vi "ConvertDtoY.vi"(8 "error in":errorcluster, 10 "Wiring Configuration":string, 11 "voltage waveform":waveform(dbl)[](array[waveform])) -> (0 "error out":errorcluster, 3 "phase voltage waveform":waveform(dbl)[](array[waveform]))   [LabVIEW 2017, in "McsaAnalysisFunctions.lvlib"]
uses:
  <vilib>/addons/InsightCM/Utilities/Analysis/MCSA/McsaAnalysisFunctions.lvlib
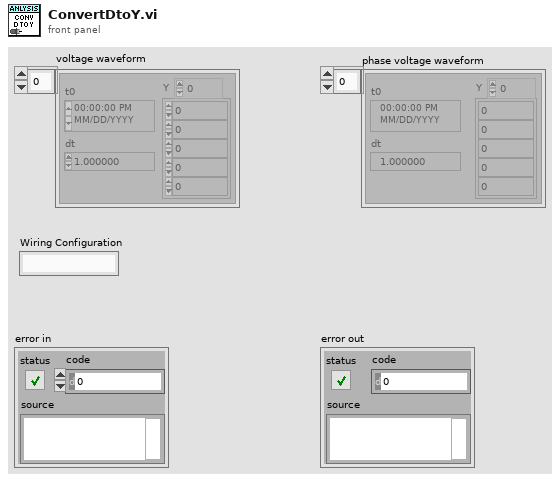
[diagram p1: front panel]
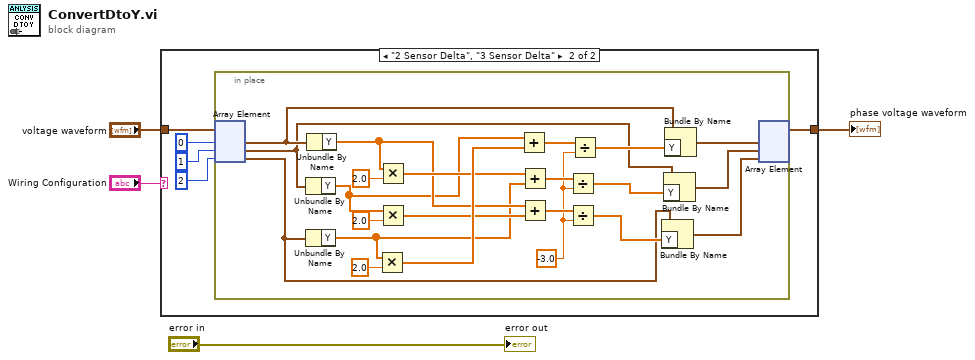
[diagram p0: block diagram]
diagram:
  n1 = case shown="\"2 Sensor Delta\", \"3 Sensor Delta\"" "Wiring Configuration" {
    tunnel: "voltage waveform" -> [w5 w10]
    tunnel: [w5 w9] -> w4
    frame "2 Sensor Wye", "3 Sensor Wye", Default {
    }
    frame "2 Sensor Delta", "3 Sensor Delta" {
      n2 = in-place {
        w17 = -3.0 ("y")
        n3 = in-place-array #1(w10, 0, 1, 2) -> (w16:waveform(dbl), w15:waveform(dbl), w14:waveform(dbl))
        n4 = Unbundle By Name(w15) -> ("Y"=w25:dbl[])
        n5 = Unbundle By Name(w14) -> ("Y"=w24:dbl[])
        n6 = Unbundle By Name(w16) -> ("Y"=w26:dbl[])
        n7 = Multiply(x=w24, y=2.0) -> (x*y=w29:dbl[])
        n8 = Multiply(x=w26, y=2.0) -> (x*y=w28:dbl[])
        n9 = Multiply(x=w25, y=2.0) -> (x*y=w27:dbl[])
        n10 = Add(x=w25, y=w29) -> (x+y=w23:dbl[])
        n11 = Add(x=w28, y=w24) -> (x+y=w22:dbl[])
        n12 = Add(x=w26, y=w27) -> (x+y=w21:dbl[])
        n13 = Divide(x=w22, y=w17) -> (x/y=w19:dbl[])
        n14 = Divide(x=w21, y=w17) -> (x/y=w18:dbl[])
        n15 = Divide(x=w23, y=w17) -> (x/y=w20:dbl[])
        n16 = Bundle By Name(cluster=w14, "Y"=w18) -> (w11:waveform(dbl))
        n17 = Bundle By Name(cluster=w15, "Y"=w19) -> (w12:waveform(dbl))
        n18 = Bundle By Name(cluster=w16, "Y"=w20) -> (w13:waveform(dbl))
        n19 = in-place-array #1(w13, w12, w11) -> (w9:waveform(dbl)[])  [unwired: 3 out]
      }
    }
  }
  "phase voltage waveform" <- w4
  "error out" <- "error in"
